vi "Lockin_Metrics.vi"() -> ()   [LabVIEW 2016]
uses:
  Instrument.Lockin/Instrument.Lockin.lvclass
  LockinDAQ/Typedefs/REF_f-array.ctl
  LockinDAQ/LockinDAQ.lvclass
  LockinDAQ/Typedefs/REF_phi-array.ctl
  LockinDAQ/Typedefs/REF-cluster.ctl
  LockinDAQ/Typedefs/AO-cluster.ctl
  LockinDAQ/Typedefs/AO_Amp-array.ctl
  LockinDAQ/Typedefs/AO_DC-array.ctl
  LockinDAQ/Typedefs/AO_phi-array.ctl
  LockinDAQ/Typedefs/Function-array.ctl
  LockinDAQ/Typedefs/Function-enum.ctl
  LockinDAQ/Typedefs/AO_f-array.ctl
panel:
  in  "Fs divisors":u32[](array[numeric])=[1, 2, 4, 8, 16]
  out "Channels: Lockin out":T1 {"REF phi (°)" format="%#_3g"}
  out "Channels: AO out":T4 {"AO f (Hz)" min=0.001 max=10000.0; "AO DC (V)" format="%.3p"; "AO Amp (V)" format="%.3p"}
  out "XY Graph":cluster{dbl[], dbl[]}[](graph)=[{[6.0, 8.0, 10.0, 13.0, 16.0, 20.0, 25.0, 32.0, 40.0, 50.0, 63.0, 79.0, 100.0, 126.0, 158.0, 200.0, 251.0, 316.0], [-1.0423552006899481, -1.3903098827137441, -1.737910087407978, -2.258602969396565, -2.780700875743044, -3.4759131475495986, -4.3427397744037775, -5.561410067975827, -6.951654879976554, -8.663719069464769, -10.951555957699167, -13.711029901411914, -17.246494034944234, -21.778009051453306, -27.24075542599655, -34.5456962508097, -43.31768132301928, -54.27310168510232]}, {[6.0, 8.0, 10.0, 13.0, 16.0, 20.0, 25.0, 32.0, 40.0, 50.0, 63.0, 79.0, 100.0, 126.0, 158.0, 200.0, 251.0, 316.0], [-2.394512524549026, -3.1951138258068474, -3.993858169174312, -5.184745780396297, -6.39037968222766, -7.988004770549838, -9.955466234078624, -12.780709734160709, -15.975883458272529, -19.821353790823995, -25.029673267394205, -31.31604215971608, -39.71735275405901, -50.22855551694198, -62.57103577930017, -79.80881797367354, -100.96616223993937, -143.65396563594373]}, {[6.0, 8.0, 10.0, 13.0, 16.0, 20.0, 25.0, 32.0, 40.0, 50.0, 63.0, 79.0, 100.0, 126.0, 158.0, 200.0, 251.0, 316.0], [-4.575602702700928, -6.105156609854453, -7.631522866632165, -9.881155067562743, -12.210535086383176, -15.263155416275039, -18.935778292399107, -24.420970742609715, -30.526174476673805, -37.93796640098544, -47.979574000445005, -59.711655402974536, -76.21887806944387, -96.51996411683551, -121.26174047622227, -153.59065300624428, 167.97792631895848, 119.38042104141758]}, {[6.0, 8.0, 10.0, 13.0, 16.0, 20.0, 25.0, 32.0, 40.0, 50.0, 63.0, 79.0, 100.0, 126.0, 158.0, 200.0, 251.0, 316.0], [-7.57964181347611, -10.13404641820485, -12.667639885328223, -16.320504761233593, -20.268332509485393, -25.335392935177406, -31.4657202920537, -40.53657512046089, -50.67071796610371, -63.16238008577377, -79.66277443157338, -100.4063846929105, -128.05440476669924, -160.22370990094828, 160.3519081985147, 107.22357024973016, 38.345551664902615, -39.56831452469504]}, {[6.0, 8.0, 10.0, 13.0, 16.0, 20.0, 25.0, 32.0, 40.0, 50.0, 63.0, 79.0, 100.0, 126.0, 158.0, 200.0, 251.0, 316.0], [-13.271355961832105, -17.741847765130448, -22.177434155746315, -28.647526806703006, -35.483952775683804, -44.35492429666974, -55.236018791420086, -70.96784186451556, -88.70976975129923, -111.98836517715236, -140.66909770193755, -175.26530770826307, 141.97077179370692, 78.63856654833467, 9.403374075159826, -84.79451570950859, 152.26167405559266, 10.325496543692617]}]
  in  "step":dbl=0.1
  in  "end":dbl=2.5
  in  "start":dbl=0.8
  in  "Channels: AO in":T4 {"AO f (Hz)" min=0.001 max=10000.0; "AO DC (V)" format="%.3p"; "AO Amp (V)" format="%.3p"}
  in  "Channels: Lockin in":T1 {"REF phi (°)" format="%#_3g"}
  # "Change the sampling frequency:"
  # "Sweep frequency:"
  # "1"
  # "2"
  # "3"
  # "4"
  # "5"
  # "6"
  # "7"
  # "8"
  # "1"
  # "2"
  # "3"
  # "4"
  # "5"
  # "6"
  # "7"
  # "8"
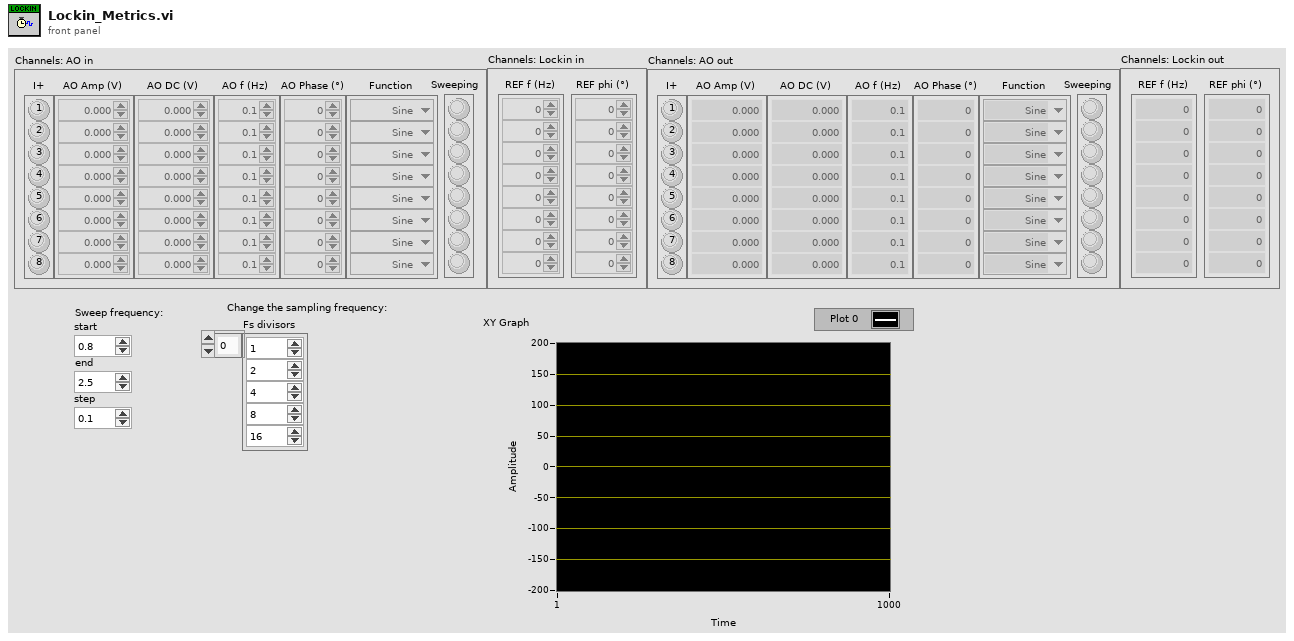
[diagram p1: front panel]
types:
  T1 = typedef "LockinDAQ.lvclass/REF-cluster.ctl" = cluster{"REF f (Hz)":T2, "REF phi (°)":T3}
  T2 = typedef "LockinDAQ.lvclass/REF_f-array.ctl" = dbl[]
  T3 = typedef "LockinDAQ.lvclass/REF_phi-array.ctl" = dbl[]
  T4 = typedef "LockinDAQ.lvclass/AO-cluster.ctl" = cluster{"AO Amp (V)":T5, "AO DC (V)":T6, "AO f (Hz)":T7, "AO Phase (°)":T8, "Function":T9, "I+":bool[], "Sweeping":bool[]}
  T5 = typedef "LockinDAQ.lvclass/AO_Amp-array.ctl" = dbl[]
  T6 = typedef "LockinDAQ.lvclass/AO_DC-array.ctl" = dbl[]
  T7 = typedef "LockinDAQ.lvclass/AO_f-array.ctl" = dbl[]
  T8 = typedef "LockinDAQ.lvclass/AO_phi-array.ctl" = dbl[]
  T9 = typedef "LockinDAQ.lvclass/Function-array.ctl" = T10[]
  T10 = typedef "LockinDAQ.lvclass/Function-enum.ctl" = enum16{"Sine", "Triangle", "Square", "Sawtooth"}
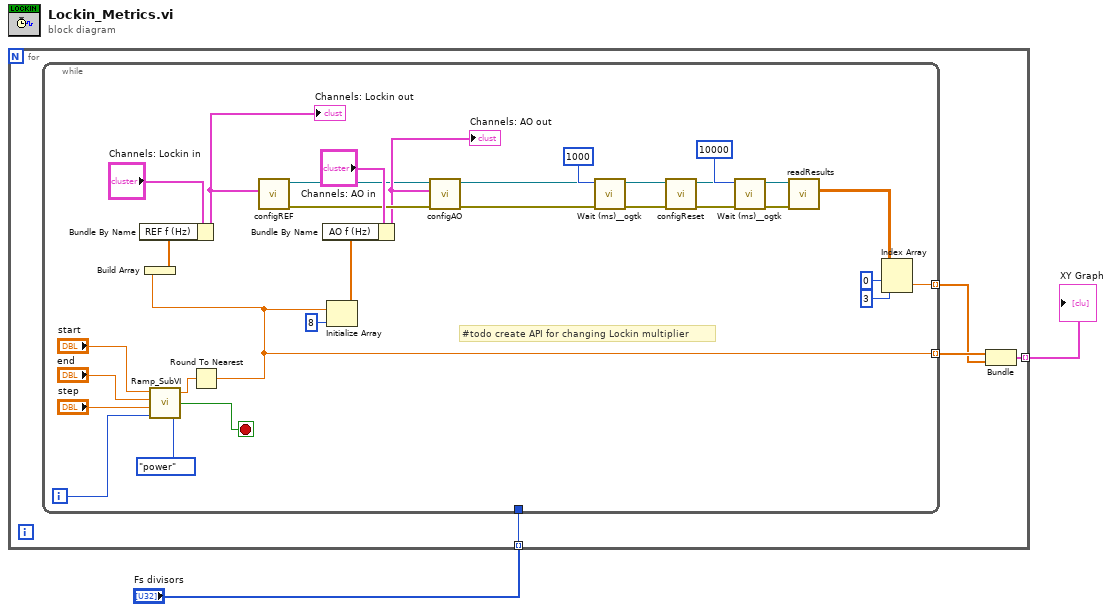
[diagram p0: block diagram]
diagram:
  n1 = for {
    tunnel: [w4] -> w1 mode=indexing
    tunnel: "Fs divisors" -> [w3] mode=indexing
    n2 = while {
      tunnel: [w13] -> w6 mode=indexing
      tunnel: [w21] -> w5 mode=indexing
      tunnel: w3 -> [_]
      i -> [w35]
      stop <- w30 stop-if-true
      # "#todo create API for changing Lockin multiplier"
      n3 = call <userlib>:"Ramp_SubVI.vi"("Enum"=enum16{"linear", "power"}."power", "index"=w35, "step"="step", "end"="end", "start"="start") -> ("Stop?"=w30:bool, "Numeric"=w26:dbl)
      n4 = Round To Nearest(number=w26) -> (nearest integer value=w13:dbl)
      n5 = Build Array(w13) -> (w27:dbl[])
      n6 = Bundle By Name(cluster="Channels: Lockin in", "REF f (Hz)"=w27) -> (w11:T1)
      "Channels: Lockin out" <- w11
      n7 = call "configREF.vi"("Channels: Lockin in"=w11) -> ("error out"=w17:errorcluster, "Instrument.Lockin out"=w9:refnum<class "Instrument.Lockin.lvclass">)  [unwired: 9 in]
      n8 = Initialize Array(w13, 8 ("dimension size")) -> (w24:dbl[])
      n9 = Bundle By Name(cluster="Channels: AO in", "AO f (Hz)"=w24) -> (w10:T4)
      "Channels: AO out" <- w10
      n10 = call "configAO.vi"("error in (no error)"=w17, "Channels: AO"=w10, "Instrument.Lockin in"=w9) -> ("error out"=w14:errorcluster, "Instrument.Lockin out"=w8:refnum<class "Instrument.Lockin.lvclass">)  [unwired: 7 in]
      n11 = call <userlib>:"Wait (ms)__ogtk.vi"("error in (no error)"=w14, "milliseconds to wait"=u32 1000) -> ("error out"=w16:errorcluster)  [unwired: 8 in, 1 out]
      n12 = call "configReset.vi"("error in (no error)"=w16, "Instrument.Lockin in"=w8) -> ("error out"=w15:errorcluster, "Instrument.Lockin out"=w7:refnum<class "Instrument.Lockin.lvclass">)  [unwired: 8 in]
      n13 = call <userlib>:"Wait (ms)__ogtk.vi"("error in (no error)"=w15, "milliseconds to wait"=u32 10000) -> ("error out"=w20:errorcluster)  [unwired: 8 in, 1 out]
      n14 = call "readResults.vi"("error in (no error)"=w20, "Instrument.Lockin in"=w7) -> ("Results"=w12:dbl[][])  [unwired: 6 in, 3 out]
      n15 = Index Array(array=w12, index (row)=0, index (col)=3 ("disabled index (col)")) -> (element=w21:dbl)
    }
    n16 = Bundle(w6, w5) -> (w4:cluster{dbl[], dbl[]})  [unwired: 1 in]
  }
  "XY Graph" <- w1
